vi "主动发送数据生成Condition(子VI).vi"(7 "结束时间":timestamp, 8 "数据发送协议":enum16{"2005-212协议", "2017-212协议"}(ring)=enum."2017-212协议", 9 "database":string, 10 "Label.Text":string, 11 "数值":i32) -> (2 "columns":string[](array[string])=["时间", "测量模式", "数据类型", "检测值", "单位", "数据标识"], 3 "CONDITION":string)   [LabVIEW 2016, in "数据传输系统.lvlib"]
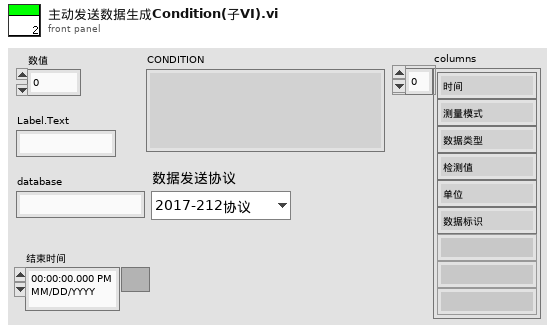
[diagram p1: front panel]
types:
  T1 = cluster{"time1":string, "time2":string, "time3":string, "time4":string, "time5":string, "time6":string, "time7":string, "time8":string, "time9":string, "time10":string, "time11":string, "time12":string, "time13":string, "time14":string, "time15":string, "time16":string, "time17":string, "time18":string, "time19":string, "time20":string, "time21":string, "time22":string, "time23":string, "time24":string, "time25":string, "time26":string, "time27":string, "time28":string, "time29":string, "time30":string, "time31":string, "time32":string, "time33":string, "time34":string, "time35":string}
  T2 = typedef "LVDateTimeRec.ctl" = cluster{"秒数的小数部分":dbl, "秒":i32, "分":i32, "时":i32, "日":i32, "月":i32, "年":i32, "天数（周）":i32, "天数（年）":i32, "DST":i32}
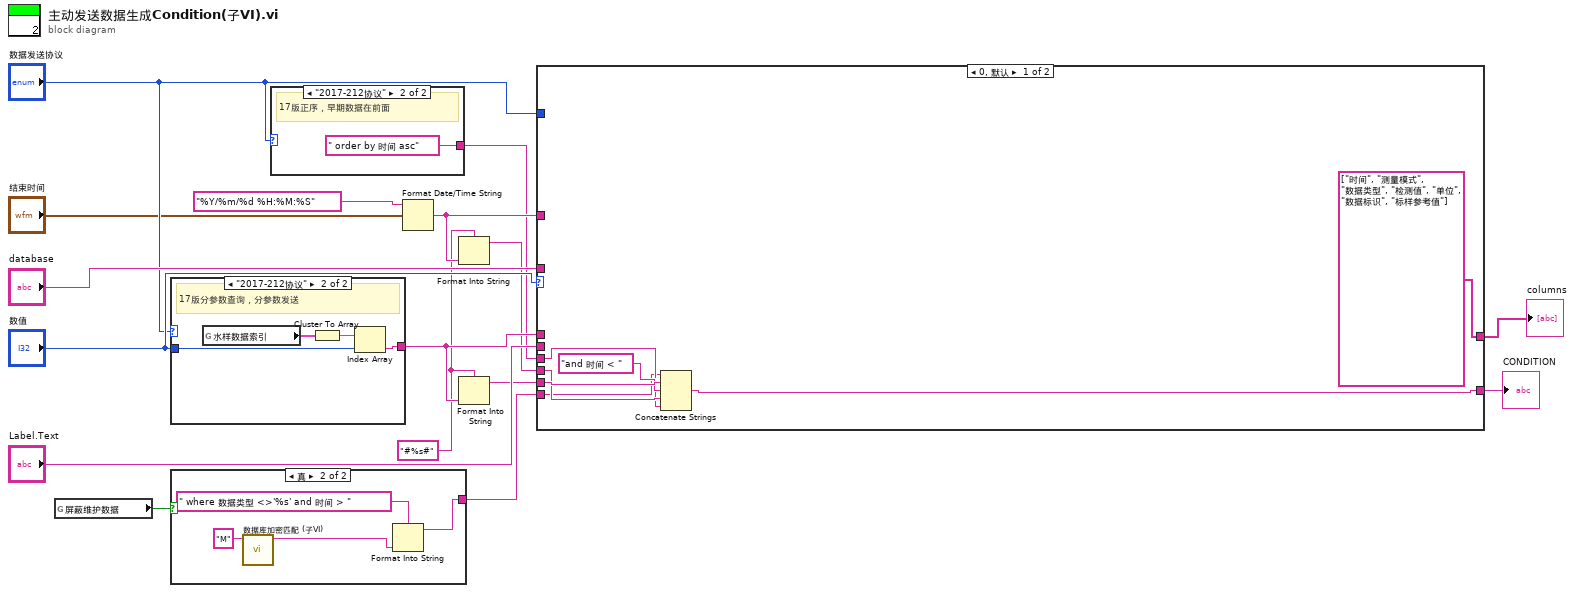
[diagram p0: block diagram]
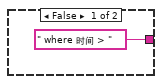
[diagram p2: hidden frame]
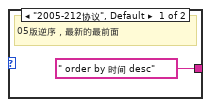
[diagram p3: hidden frame]
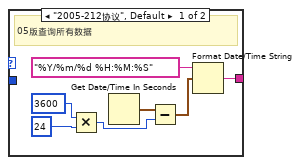
[diagram p4: hidden frame]
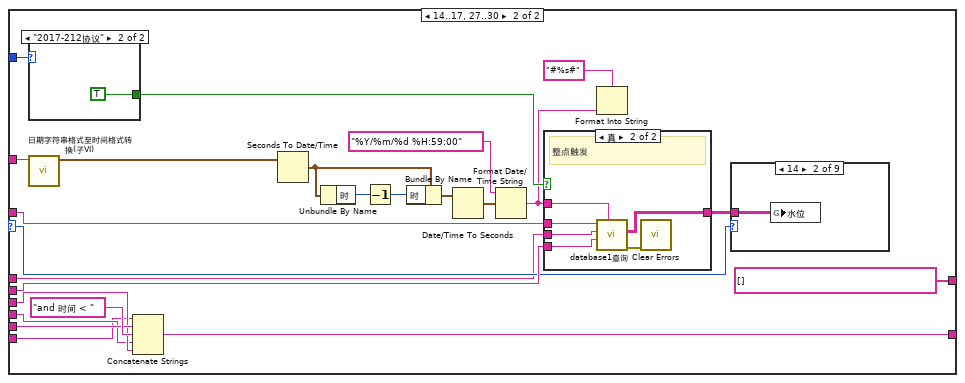
[diagram p5: hidden frame]
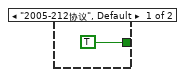
[diagram p6: hidden frame]
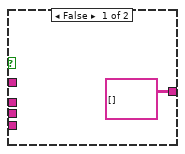
[diagram p7: hidden frame]
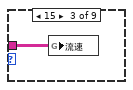
[diagram p9: hidden frame]
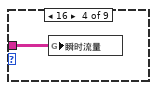
[diagram p10: hidden frame]
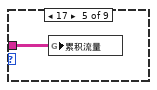
[diagram p11: hidden frame]
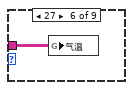
[diagram p12: hidden frame]
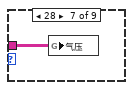
[diagram p13: hidden frame]
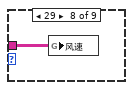
[diagram p14: hidden frame]
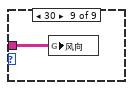
[diagram p15: hidden frame]
diagram:
  w3 = "#%s#" ("初始字符串")
  n1 = global read "断电保存全局.vi" "屏蔽维护数据"() -> (w1:bool)
  n2 = case shown="\"2017-212协议\"" "数据发送协议" {
    tunnel: [w22 w24] -> w15
    tunnel: "数值" -> [_ w25]
    frame "2005-212协议", Default {
      # "05版查询所有数据"
      n3 = Multiply(x=3600, y=24) -> (x*y=w17:i32)
      n4 = Get Date/Time In Seconds() -> (seconds since 1Jan1904=w21:timestamp)
      n5 = Subtract(x=w21, y=w17) -> (x-y=w20:timestamp)
      n6 = Format Date/Time String(time format string (%c)="%Y/%m/%d %H:%M:%S" ("时间格式字符串(%c)"), seconds (now)=w20) -> (date/time string=w22:string)  [unwired: 1 in]
    }
    frame "2017-212协议" {
      # "17版分参数查询，分参数发送"
      n7 = global read "全局 水样时间.vi" "水样数据索引"() -> (w26:T1)
      n8 = Cluster To Array(cluster=w26) -> (array=w27:string[])
      n9 = Index Array(array=w27, index=w25) -> (element=w24:string)
    }
  }
  n10 = case shown="真" w1 {
    tunnel: [" where 时间 > " w31] -> w2
    frame False {
    }
    frame True {
      n11 = call "数据库加密匹配 (子VI).vi"("输入参数"="M") -> ("Encoded String"=w29:string)  [unwired: 10 in]
      n12 = Format Into String(format string=" where 数据类型 <>'%s' and 时间 > ", w29) -> (resulting string=w31:string)  [unwired: 2 in, 1 out]
    }
  }
  n13 = case shown="\"2017-212协议\"" "数据发送协议" {
    tunnel: [" order by 时间 desc" ("字符串") " order by 时间 asc" ("字符串")] -> w9
    frame "2005-212协议", Default {
      # "05版逆序，最新的最前面"
    }
    frame "2017-212协议" {
      # "17版正序，早期数据在前面"
    }
  }
  n14 = Format Date/Time String(time format string (%c)="%Y/%m/%d %H:%M:%S" ("时间格式字符串(%c)"), seconds (now)="结束时间") -> (date/time string=w16:string)  [unwired: 1 in]
  n15 = Format Into String(format string=w3, w16) -> (resulting string=w11:string)  [unwired: 2 in, 1 out]
  n16 = Format Into String(format string=w3, w15) -> (resulting string=w10:string)  [unwired: 2 in, 1 out]
  n17 = case shown="0, 默认" "数值" {
    selector: "数值" -> [_ w59]
    tunnel: w10 -> [w41 w63]
    tunnel: [w40 w64] -> w5
    tunnel: w11 -> [w38 w44]
    tunnel: "database" -> [_ w62]
    tunnel: "Label.Text" -> [_ w61]
    tunnel: w15 -> [_ w43]
    tunnel: w16 -> [_ w47]
    tunnel: w9 -> [w37 w58]
    tunnel: [string[] ["时间", "测量模式", "数据类型", "检测值", "单位", "数据标识", "标样参考值"] ("columns") string[] [] ("columns")] -> w8
    tunnel: "数据发送协议" -> [_ w55]
    tunnel: w2 -> [w35 w42]
    frame 0, Default {
      n18 = Concatenate Strings(w35, w41, "and 时间 < " ("字符串"), w38, w37) -> (w40:string)
    }
    frame 14..17, 27..30 {
      n19 = case shown="\"2017-212协议\"" w55 {
        tunnel: [TRUE TRUE] -> w57
        frame "2005-212协议", Default {
        }
        frame "2017-212协议" {
        }
      }
      n20 = call "日期字符串格式至时间格式转换(子VI).vi"("data[0]"=w47) -> ("time stamp"=w50:timestamp)  [unwired: 10 in]
      n21 = Concatenate Strings(w42, w63, "and 时间 < " ("字符串"), w44, w58) -> (w64:string)
      n22 = Seconds To Date/Time(time stamp (now)=w50) -> (date time rec=w52:T2)  [unwired: 1 in]
      n23 = Unbundle By Name(w52) -> ("时"=w53:i32)
      n24 = Decrement(x=w53) -> (x-1=w54:i32)
      n25 = Bundle By Name(cluster=w52, "时"=w54) -> (w51:T2)
      n26 = Date/Time To Seconds(2:w51) -> (0:w49:timestamp)  [unwired: 1 in]
      n27 = Format Date/Time String(time format string (%c)="%Y/%m/%d %H:59:00" ("时间格式字符串(%c)"), seconds (now)=w49) -> (date/time string=w45:string)  [unwired: 1 in]
      n28 = case shown="真" w57 {
        tunnel: w62 -> [_ w74]
        tunnel: w61 -> [_ w73]
        tunnel: [string[][] [] ("data") w72] -> w60
        tunnel: w45 -> [_ w71]
        tunnel: w43 -> [_ w69]
        frame False {
        }
        frame True {
          # "整点触发"
          n29 = call "database1查询.vi"("时间2"=w71, "table"=w73, "时间1"=w69, "database"=w74) -> ("error out"=w70:errorcluster, "data"=w72:string[][])  [unwired: 4 in, 1 out]
          n30 = call <vilib>:"Clear Errors.vi"("error in (no error)"=w70) -> ()  [unwired: 5 in, 2 out]
        }
      }
      n31 = Format Into String(format string="#%s#" ("初始字符串"), w45) -> ()  [unwired: 2 in, 2 out]
      n32 = case shown="14" w59 {
        tunnel: w60 -> [_ w75 w76 w77 w78 w79 w80 w81 w82]
        frame 0, Default {
        }
        frame 14 {
          n33 = global write "全局 所有参数.vi" "水位"(w75) -> ()
        }
        frame 15 {
          n34 = global write "全局 所有参数.vi" "流速"(w76) -> ()
        }
        frame 16 {
          n35 = global write "全局 所有参数.vi" "瞬时流量"(w77) -> ()
        }
        frame 17 {
          n36 = global write "全局 所有参数.vi" "累积流量"(w78) -> ()
        }
        frame 27 {
          n37 = global write "全局 所有参数.vi" "气温"(w79) -> ()
        }
        frame 28 {
          n38 = global write "全局 所有参数.vi" "气压"(w80) -> ()
        }
        frame 29 {
          n39 = global write "全局 所有参数.vi" "风速"(w81) -> ()
        }
        frame 30 {
          n40 = global write "全局 所有参数.vi" "风向"(w82) -> ()
        }
      }
    }
  }
  "CONDITION" <- w5
  "columns" <- w8
